vi "Multiply and Add using DSP48E.vi"() -> ()   [LabVIEW 2011]
uses:
  <vilib>/rvi/FXPMathLib/FxpConvert/subVIs/nifxpmath_Convert_SimConfig.ctl
  <vilib>/fxp/LVFixedPointQuantizationPolicyTypeDef.ctl
  <vilib>/fxp/LVFixedPointOverflowPolicyTypeDef.ctl
  <vilib>/rvi/FXPMathLib/basic elements/DSP48E/simVIs/niFpgaDsp48eRegisters.ctl
  <vilib>/rvi/FXPMathLib/basic elements/DSP48E/simVIs/niFpgaDsp48eEnables.ctl
  <vilib>/rvi/FXPMathLib/basic elements/DSP48E/simVIs/niFpgaDsp48eResets.ctl
  <vilib>/rvi/FXPMathLib/basic elements/DSP48E/simVIs/niFpgaDsp48eSimulationState.ctl
  <vilib>/rvi/FXPMathLib/basic elements/DSP48E/subVIs/niFpgaDsp48eType.ctl
  <vilib>/rvi/FXPMathLib/basic elements/DSP48E/subVIs/niFpgaDsp48eAlumodeOpmodeCarryinselState.ctl
  <vilib>/rvi/FXPMathLib/basic elements/DSP48E/subVIs/niFpgaDsp48eUseMultiplierState.ctl
  <vilib>/rvi/FXPMathLib/basic elements/DSP48E/subVIs/niFpgaDsp48eLogicUnitModeState.ctl
  <vilib>/rvi/FXPMathLib/basic elements/DSP48E/subVIs/niFpgaDsp48eSelectPatternState.ctl
  <vilib>/rvi/FXPMathLib/basic elements/DSP48E/subVIs/niFpgaDsp48eSelectMaskState.ctl
  <vilib>/rvi/FXPMathLib/basic elements/DSP48E/subVIs/niFpgaDsp48eAutoresetState.ctl
  <vilib>/rvi/FXPMathLib/FxpConvert/simVIs/DllFxpConvertTemp_sub.vi
  <vilib>/rvi/FXPMathLib/basic elements/DSP48E/simVIs/niFpgaDsp48eSimMultiplier.vi
  <vilib>/rvi/FXPMathLib/basic elements/DSP48E/simVIs/niFpgaDsp48eSimArithmetic.vi
  <vilib>/rvi/FXPMathLib/basic elements/DSP48E/simVIs/niFpgaDsp48eSimPatternDetect.vi
  <vilib>/rvi/FXPMathLib/basic elements/DSP48E/simVIs/niFpgaDsp48eSimP.vi
  <vilib>/rvi/FXPMathLib/basic elements/DSP48E/simVIs/niFpgaDsp48eSimUpdateState.vi
  <vilib>/rvi/FXPMathLib/basic elements/DSP48E/simVIs/niFpgaDsp48eCheckMode.vi
  <vilib>/rvi/FXPMathLib/basic elements/DSP48E/simVIs/niFpgaDsp48eReportInvalidMode.vi
  <vilib>/rvi/FXPMathLib/FxpInterpret/XNode/nifxpmath_Interpret.xnode
  <vilib>/rvi/FXPMathLib/FxpConvert/XNode/nifxpmath_Convert.xnode
  <vilib>/rvi/FXPMathLib/basic elements/DSP48E/XNode/niFpgaDsp48e.xnode
panel:
  out "a*b+c":fxp<+/-,48,16> format="%.37g"
  in  "c":fxp<+/-,16,1> format="%.6f"
  in  "b":fxp<+/-,18,1>
  in  "a":fxp<+/-,16,1> format="%.6f"
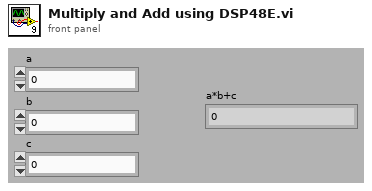
[diagram p1: front panel]
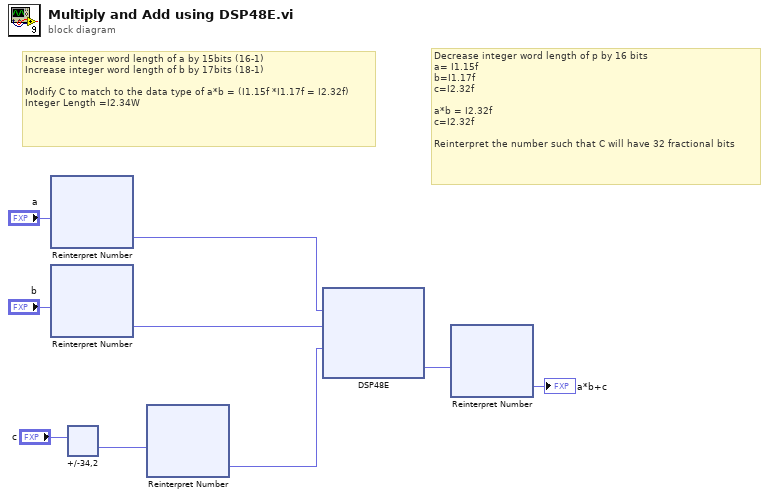
[diagram p0: block diagram]
diagram:
  # "Decrease integer word length of p by 16 bits\na= I1.15f\nb=I1.17f\nc=I2.32f\n\na*b = I2.32f\nc=I2.32f\n\nReinterpret the number such that C will have 32 fractional bits"
  # "Increase integer word length of a by 15bits (16-1)\nIncrease integer word length of b by 17bits (18-1)\n\nModify C to match to the data type of a*b = (I1.15f *I1.17f = I2.32f)\nInteger Length =I2.34W"
  n1 = xnode "Reinterpret Number"("x"="a") -> ("y"=w4:fxp<+/-,16,16>)
  n2 = xnode "Reinterpret Number"("x"="b") -> ("y"=w7:fxp<+/-,18,18>)
  n3 = xnode "+/-34,2"("x"="c") -> ("y"=w1:fxp<+/-,34,2>)
  n4 = xnode "Reinterpret Number"("x"=w1) -> ("y"=w3:fxp<+/-,34,34>)
  n5 = xnode "DSP48E"("a"=w4, "b"=w7, "c"=w3) -> ("p"=w6:fxp<+/-,48,48>)
  n6 = xnode "Reinterpret Number"("x"=w6) -> ("y"=→"a*b+c":fxp<+/-,48,16>)
